vi "Logic.vi"(8 "error in (no error)":errorcluster, 11 "CIFTemplatePlugin in":refnum<class "Template_Plugin.lvclass">) -> (0 "error out":errorcluster, 3 "CIFTemplatePlugin out":refnum<class "Template_Plugin.lvclass">)   [LabVIEW 2021, in "Template_Plugin.lvclass"]
uses:
  Template_Plugin.lvclass
  Template_Plugin.lvclass/Template_Plugin.ctl
  <vilib>/CIF Foundation/CIF Core/CIFCore/Class/CIFCorePlugin.lvclass
  Common/Typedef/Channels.ctl
  Common/Template_Common.lvlib
  C:/Program Files/National Instruments/LabVIEW 2021/vi.lib/CIF Foundation/CIF Core/CIFCore/Class/CIFCorePlugin.lvclass
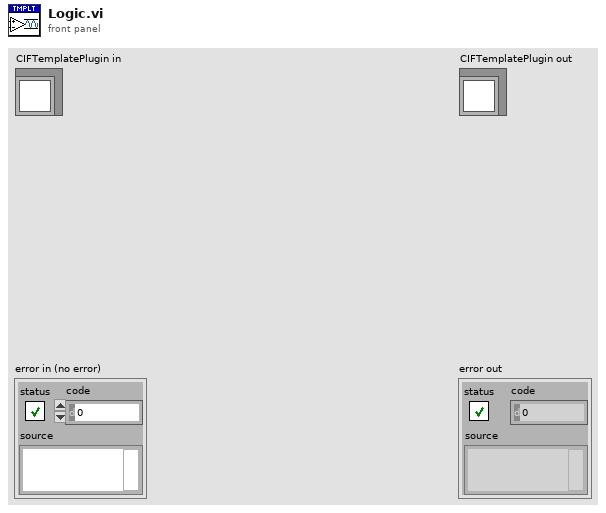
[diagram p1: front panel]
types:
  T1 = typedef "Template_Common.lvlib/Channels.ctl" = enum16{"doubleout", "doublein1", "doublein2", "uint_out", "uint_in", "u8array_out", "u8array_in"}
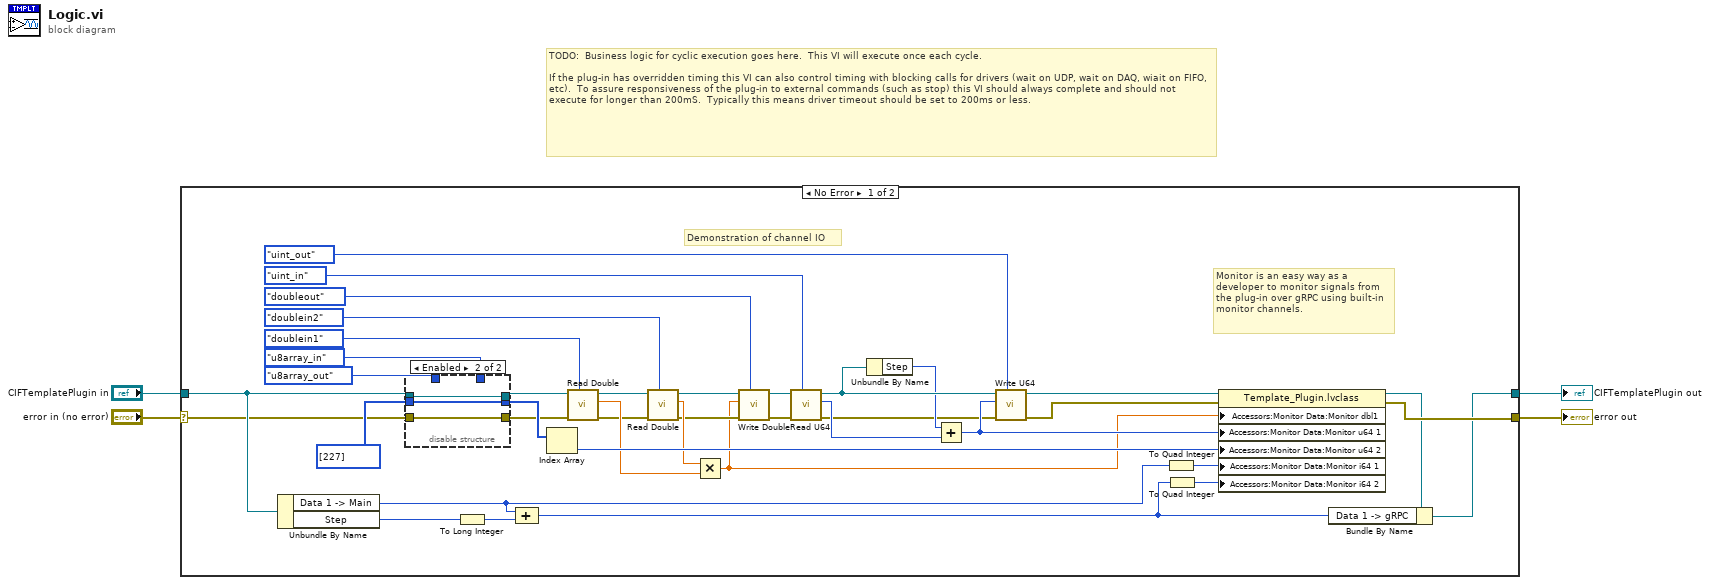
[diagram p0: block diagram]
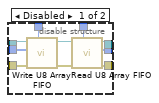
[diagram p2: hidden frame]
diagram:
  # "TODO:  Business logic for cyclic execution goes here.  This VI will execute once each cycle.  \n\nIf the plug-in has overridden timing this VI can also control timing with blocking calls for drivers (wait on UDP, wait on DAQ, wiait on FIFO, etc).  To assure responsiveness of the plug-in to external commands (such as stop) this VI should always complete and should not execute for longer than 200mS.  Typically this means driver timeout should be set to 200ms or less."
  n1 = case shown="No Error" "error in (no error)" {
    selector: "error in (no error)" -> [w6 w58]
    tunnel: [w43 w58] -> w2
    tunnel: [w35 w57] -> w1
    tunnel: "CIFTemplatePlugin in" -> [w27 w57]
    frame No Error {
      # "Demonstration of channel IO"
      # "Monitor is an easy way as a developer to monitor signals from the plug-in over gRPC using built-in monitor channels."
      n2 = Unbundle By Name(w27) -> ("Data 1 -> Main"=w40:i32, "Step"=w33:u64)
      n3 = disable-structure shown="Enabled" {
        disable-tunnel: w27 -> [w53 w56]
        disable-tunnel: Channels."u8array_out" ("Channels") -> [w52 _]
        disable-tunnel: u8[] [227] ("Data in") -> [w51 w54]
        disable-tunnel: Channels."u8array_in" ("Channels") -> [w49 _]
        disable-tunnel: [w48 w54] -> w23
        disable-tunnel: [w47 w56] -> w19
        disable-tunnel: [w46 w55] -> w7
        disable-tunnel: w6 -> [w44 w55]
        frame Disabled {
          n4 = call <vilib>:"Write U8 Array FIFO.vi"("Channel Index"=w52, "error in (no error)"=w44, "Data"=w51, "CIFCorePlugin in"=w53) -> ("error out"=w45:errorcluster, "CIFCorePlugin in"=w50:refnum<class "Template_Plugin.lvclass">)  [unwired: 5 in, 1 out]
          n5 = call <vilib>:"Read U8 Array FIFO.vi"("Channel Index"=w49, "error in (no error)"=w45, "CIFCorePlugin in"=w50) -> ("error out"=w46:errorcluster, "Data"=w48:u8[], "CIFCorePlugin in"=w47:refnum<class "Template_Plugin.lvclass">)  [unwired: 4 in, 2 out]
        }
        frame Enabled {
        }
      }
      n6 = To Long Integer(number=w33) -> (32bit integer=w41:i32)
      n7 = Compound Arithmetic op=ADD(w40, w41) -> (w39:i32)
      n8 = Index Array(array=w23) -> (element=w28:u8)  [unwired: 1 in]
      n9 = call <vilib>:"Read Double.vi"("Channel Index"=Channels."doublein1" ("Channels"), "error in (no error)"=w7, "CIFCorePlugin in"=w19) -> ("error out"=w17:errorcluster, "Data"=w18:dbl, "CIFCorePlugin in"=w16:refnum<class "Template_Plugin.lvclass">)  [unwired: 6 in]
      n10 = call <vilib>:"Read Double.vi"("Channel Index"=Channels."doublein2" ("Channels"), "error in (no error)"=w17, "CIFCorePlugin in"=w16) -> ("error out"=w14:errorcluster, "Data"=w15:dbl, "CIFCorePlugin in"=w13:refnum<class "Template_Plugin.lvclass">)  [unwired: 6 in]
      n11 = Multiply(x=w15, y=w18) -> (x*y=w12:dbl)
      n12 = call <vilib>:"Write Double.vi"("Channel Index"=Channels."doubleout" ("Channels"), "error in (no error)"=w14, "Data"=w12, "CIFCorePlugin in"=w13) -> ("error out"=w10:errorcluster, "CIFCorePlugin in"=w11:refnum<class "Template_Plugin.lvclass">)  [unwired: 6 in]
      n13 = call <vilib>:"Read U64.vi"("Channel Index"=Channels."uint_in" ("Channels"), "error in (no error)"=w10, "CIFCorePlugin in"=w11) -> ("error out"=w8:errorcluster, "Data"=w31:u64, "CIFCorePlugin in"=w32:refnum<class "Template_Plugin.lvclass">)  [unwired: 6 in]
      n14 = Unbundle By Name(w32) -> ("Step"=w30:u64)
      n15 = Add(x=w30, y=w31) -> (x+y=w29:u64)
      n16 = call <vilib>:"Write U64.vi"("Channel Index"=Channels."uint_out" ("Channels"), "error in (no error)"=w8, "Data"=w29, "CIFCorePlugin in"=w32) -> ("error out"=w9:errorcluster, "CIFCorePlugin in"=w5:refnum<class "Template_Plugin.lvclass">)  [unwired: 6 in]
      n17 = To Quad Integer(1:w40) -> (0:w38:i64)
      n18 = To Quad Integer(1:w39) -> (0:w37:i64)
      n19 = property class="Template_Plugin.lvclass"(reference=w5, error in=w9, "Accessors:Monitor Data:Monitor dbl1"=w12, "Accessors:Monitor Data:Monitor u64 1"=w29, "Accessors:Monitor Data:Monitor u64 2"=w28, "Accessors:Monitor Data:Monitor i64 1"=w38, "Accessors:Monitor Data:Monitor i64 2"=w37) -> (reference out=w36:refnum<class "Template_Plugin.lvclass">, error out=w43:errorcluster)
      n20 = Bundle By Name(cluster=w36, "Data 1 -> gRPC"=w39) -> (w35:refnum<class "Template_Plugin.lvclass">)
    }
    frame Error {
    }
  }
  "error out" <- w2
  "CIFTemplatePlugin out" <- w1
